vi "get_subset.vi"(7 "retrieval mode":T1, 8 "error in (no error)":errorcluster, 9 "min (x/y/z)":dbl[](array[numeric]), 10 "max (x/y/z)":dbl[](array[numeric]), 11 "PointCollection in":refnum<class "PointCollection.lvclass">) -> (0 "error out":errorcluster, 2 "points":dbl[][](array[numeric]), 3 "PointCollection out":refnum<class "PointCollection.lvclass">)   [LabVIEW 2010, in "PointCollection.lvclass"]
uses:
  PointCollection.lvclass
  mode_enum.ctl
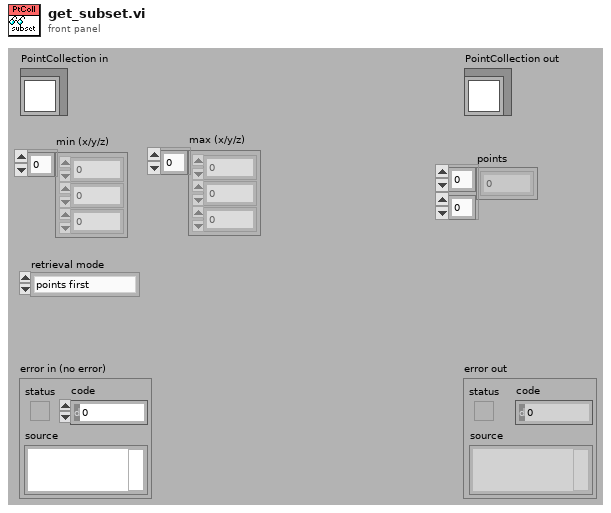
[diagram p1: front panel]
types:
  T1 = typedef "PointCollection.lvclass/mode_enum.ctl" = enum16{"points first", "dimensions first"}
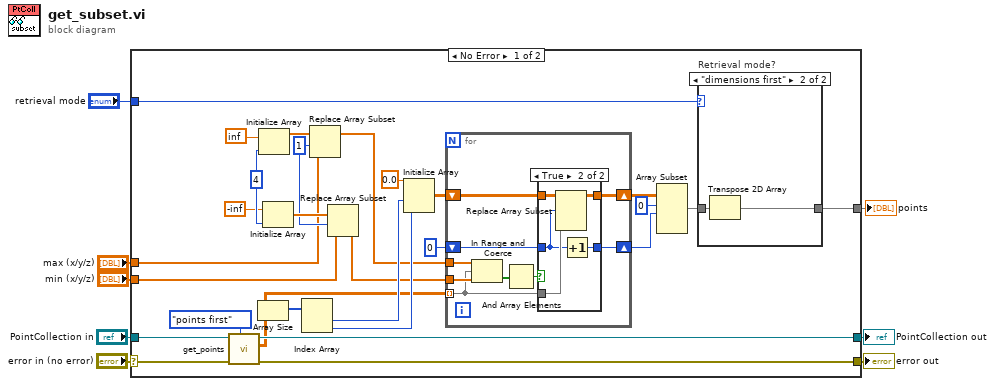
[diagram p0: block diagram]
diagram:
  n1 = case shown="No Error" "error in (no error)" {
    selector: "error in (no error)" -> [w32 w57]
    tunnel: [w36 w57] -> w7
    tunnel: [w35 w56] -> w5
    tunnel: "PointCollection in" -> [w31 w56]
    tunnel: "max (x/y/z)" -> [w17 _]
    tunnel: "min (x/y/z)" -> [w16 _]
    tunnel: "retrieval mode" -> [w11 _]
    tunnel: [w9 _] -> w1
    frame No Error {
      w18 = 1 ("index")
      w21 = 4 ("y")
      n2 = call-dynamic "get_points.vi"("retrieval mode"=mode_enum."points first", "error in (no error)"=w32, "PointCollection in"=w31) -> ("error out"=w36:errorcluster, "points"=w25:dbl[][], "PointCollection out"=w35:refnum<class "PointCollection.lvclass">)  [unwired: 6 in]
      n3 = Array Size(array=w25) -> (size(s)=w30:i32[])
      n4 = Initialize Array(inf, w21) -> (w20:dbl[])
      n5 = Initialize Array(-inf, w21) -> (w19:dbl[])
      n6 = Index Array(array=w30) -> (element #1=w29:i32, element #2=w28:i32)  [unwired: 2 in]
      n7 = Replace Array Subset(array=w20, new element=w17, index=w18) -> (w14:dbl[])
      n8 = Replace Array Subset(array=w19, new element=w16, index=w18) -> (w15:dbl[])
      n9 = Initialize Array(0.0, w29, w28) -> (w33:dbl[][])
      n10 = for {
        tunnel: w25 -> [w40] mode=indexing
        tunnel: w15 -> [w47]
        tunnel: w14 -> [w48]
        shift-right: [w43] -> w26
        shift-left: w33 -> [w46]
        shift-right: [w44] -> w24
        shift-left: 0 -> [w45]
        n11 = In Range and Coerce(upper limit=w48, x=w40, lower limit=w47) -> (In Range?=w42:bool[])  [unwired: 1 out]
        n12 = And Array Elements(Boolean array=w42) -> (logical AND=w41:bool)
        n13 = case shown="True" w41 {
          tunnel: w46 -> [w49 w55]
          tunnel: w45 -> [w50 w51]
          tunnel: [w50 w54] -> w44
          tunnel: [w49 w53] -> w43
          tunnel: w40 -> [_ w52]
          frame False {
          }
          frame True {
            n14 = Replace Array Subset(array=w55, new element=w52, index (row)=w51) -> (w53:dbl[][])  [unwired: 1 in]
            n15 = Increment(x=w51) -> (x+1=w54:i32)
          }
        }
      }
      n16 = Array Subset(array=w26, index (row)=0 ("index"), length (row)=w24) -> (w10:dbl[][])  [unwired: 2 in]
      n17 = case "Retrieval mode?" shown="\"dimensions first\"" w11 {
        tunnel: w10 -> [w37 w39]
        tunnel: [w37 w38] -> w9
        frame "points first", Default {
        }
        frame "dimensions first" {
          n18 = Transpose 2D Array(2D array=w39) -> (transposed array=w38:dbl[][])
        }
      }
    }
    frame Error {
    }
  }
  "error out" <- w7
  "PointCollection out" <- w5
  "points" <- w1
